vi "runTestScenario.vi"(0 "Constant Analog Output Voltage Test  in":refnum<class "Constant Analog Output Voltage Test.lvclass">, 5 "ILC":refnum<class "ILC.lvclass">, 11 "error in (no error)":errorcluster) -> (4 "Constant Analog Output Voltage Test  out":refnum<class "Constant Analog Output Voltage Test.lvclass">, 6 "ILC 2":refnum<class "ILC.lvclass">, 8 "TestExecution":T2, 10 "Result":T1, 15 "error out":errorcluster)   [LabVIEW 2016, in "Constant Analog Output Voltage Test.lvclass"]
uses:
  Constant Analog Output Voltage Test.lvclass
  Typedefs/TestExecution.ctl
  Typedefs/PassFailTest.ctl
  Common_ILC/ILC/ILC.lvclass
  Typedefs/WriteDataFileInput.ctl
  Typedefs/TestScenarioTypes.ctl
  Typedefs/WriteLogMessageInput.ctl
  Constant Analog Output Voltage Test.lvclass/Constant Analog Output Voltage Test.ctl
  Model/TestLog/ITestLog/ITestLog.lvclass
  Typedefs/ILCBTTypedefs.lvlib
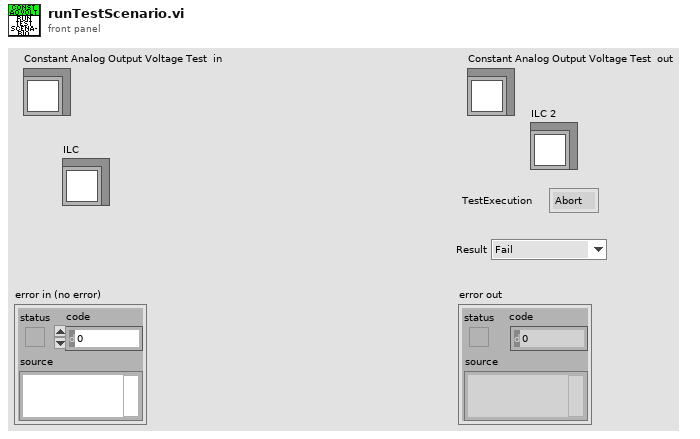
[diagram p1: front panel]
types:
  T1 = typedef "ILCBTTypedefs.lvlib/PassFailTest.ctl" = enum16{"Fail", "Pass", "NA"}
  T2 = typedef "ILCBTTypedefs.lvlib/TestExecution.ctl" = enum16{"Abort", "Continue"}
  T3 = typedef "ILCBTTypedefs.lvlib/WriteLogMessageInput.ctl" = cluster{"Test Scenario":T4, "Description":string, "Actual Value":string, "Data File":string, "Result":T1}
  T4 = typedef "ILCBTTypedefs.lvlib/TestScenarioTypes.ctl" = enum16{"+3.3VD", "+5.1V", "+24V", "RELVALV1", "RELVALV2", "Verify DAC_A = -1.00A", "Verify DAC_A = -0.75A", "Verify DAC_A = -0.50A", "Verify DAC_A = -0.25A", "Verify DAC_A = 0.00A", "Verify DAC_A = 0.25A", "Verify DAC_A = 0.50A", "Verify DAC_A = 0.75A", "Verify DAC_A = 1.00A", "Verify DAC_B = -1.00A", "Verify DAC_B = -0.75A", "Verify DAC_B = -0.50A", "Verify DAC_B = -0.25A", "Verify DAC_B = 0.00A", "Verify DAC_B = 0.25A", "Verify DAC_B = 0.50A", "Verify DAC_B = 0.75A", "Verify DAC_B = 1.00A", "Set DAC_A = -1.00A", "Set DAC_A = -0.75A", "Set DAC_A = -0.50A", "Set DAC_A = -0.25A", "Set DAC_A = 0.00A", "Set DAC_A = 0.25A", "Set DAC_A = 0.50A", "Set DAC_A = 0.75A", "Set DAC_A = 1.00A", "Set DAC_B = -1.00A", "Set DAC_B = -0.75A", "Set DAC_B = -0.50A", "Set DAC_B = -0.25A", "Set DAC_B = 0.00A", "Set DAC_B = 0.25A", "Set DAC_B = 0.50A", "Set DAC_B = 0.75A", "Set DAC_B = 1.00A", "Set MTR_PWR = On", "Set MTR_PWR = Off", "Set OUTPUT = On", "Set OUTPUT = Off", "Verify OUTPUT = On", "Verify OUTPUT = Off", "Verify POWER = Ok", "Verify POWER = Fail", "Verify AMP1 = Ok", "Verify AMP1 = Fail", "Verify AMP2 = Ok", "Verify AMP2 = Fail", "P1 0%", "P1 25%", "P1 50%", "P1 75%", "P1 100%", "P2 0%", "P2 25%", "P2 50%", "P2 75%", "P2 100%", "P3 0%", "P3 25%", "P3 50%", "P3 75%", "P3 100%", "P4 0%", "P4 25%", "P4 50%", "P4 75%", "P4 100%", "DCA 1 Linearity", "DCA 2 Linearity"}
  T5 = typedef "ILCBTTypedefs.lvlib/WriteDataFileInput.ctl" = cluster{"Test Scenario":T4, "File Name":string, "Output":string[]}
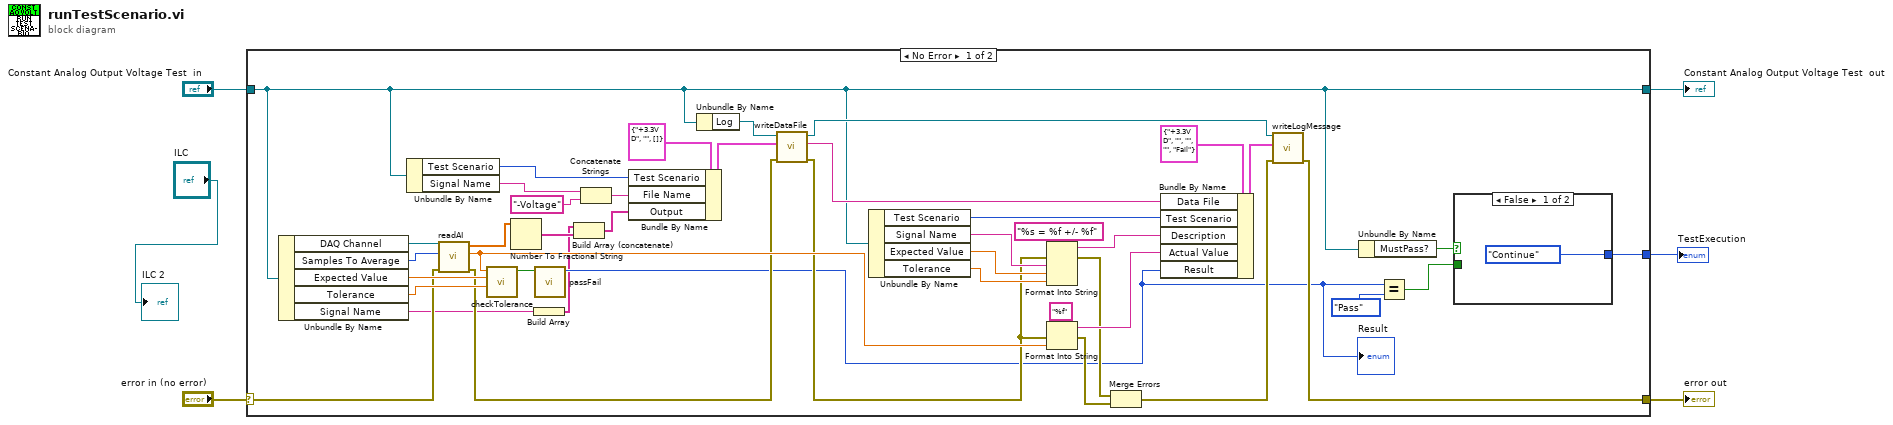
[diagram p0: block diagram]
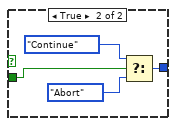
[diagram p2: hidden frame]
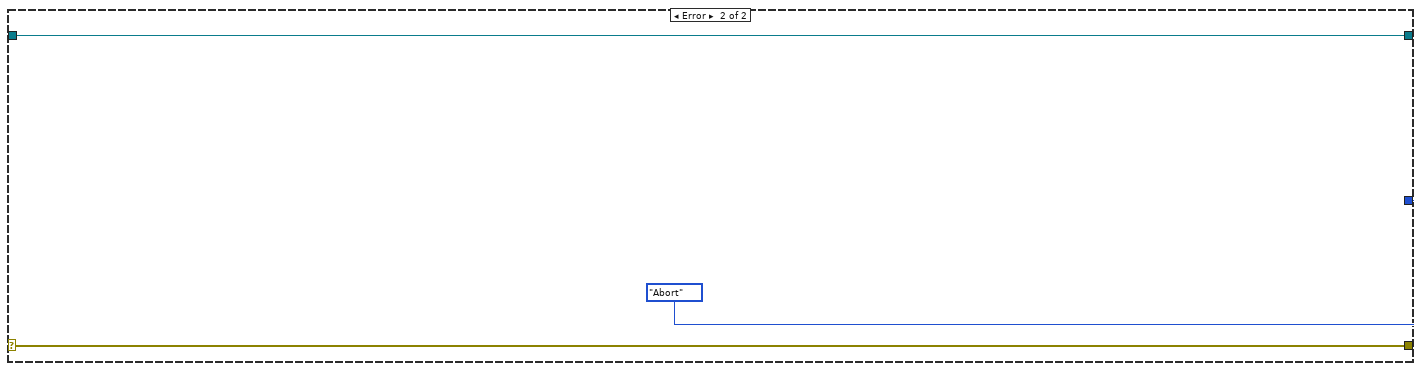
[diagram p3: hidden frame]
diagram:
  n1 = case shown="No Error" "error in (no error)" {
    selector: "error in (no error)" -> [w25 w57]
    tunnel: [w20 w57] -> w5
    tunnel: [w16 TestExecution."Abort" ("TestExecution")] -> w4
    tunnel: "Constant Analog Output Voltage Test  in" -> [w18 w55]
    tunnel: [w18 w55] -> w2
    frame No Error {
      n2 = Unbundle By Name(w18) -> ("DAQ Channel"=w49:refnum<k21>, "Samples To Average"=w42:i32, "Expected Value"=w41:dbl, "Tolerance"=w40:dbl, "Signal Name"=w8:string)
      n3 = Unbundle By Name(w18) -> ("Test Scenario"=w45:T4, "Signal Name"=w44:string)
      n4 = call "readAI.vi"("error in (no error)"=w25, "Samples To Read"=w42, "DAQ Channel To Read"=w49) -> ("error out"=w24:errorcluster, "Average"=w28:dbl, "Samples"=w13:dbl[])  [unwired: 6 in]
      n5 = call "checkTolerance.vi"("Tolerance"=w40, "Expected Value"=w41, "Average"=w28) -> ("Boolean"=w37:bool)  [unwired: 8 in]
      n6 = Number To Fractional String(number=w13) -> (F-format string=w10:string[])  [unwired: 3 in]
      n7 = Build Array(w8) -> (w7:string[])
      n8 = call "passFail.vi"("Boolean"=w37) -> ("Result"=w12:T1)  [unwired: 10 in]
      "Result" <- w12
      n9 = Build Array (concatenate)(w7, w10) -> (w9:string[])
      n10 = Concatenate Strings(w44, "-Voltage" ("string")) -> (w43:string)
      n11 = Bundle By Name(cluster=T5 {"Test Scenario"=enum."+3.3VD", "File Name"="", "Output"=[]} ("WriteDataFileInput"), "Test Scenario"=w45, "File Name"=w43, "Output"=w9) -> (w46:T5)
      n12 = Unbundle By Name(w18) -> ("Log"=w48:refnum<class "ITestLog.lvclass">)
      n13 = call-dynamic "writeDataFile.vi"("error in (no error)"=w24, "WriteDataFileInput"=w46, "ITestLog in"=w48) -> ("error out"=w19:errorcluster, "Relative Path"=w36:string, "ITestLog out"=w26:refnum<class "ITestLog.lvclass">)  [unwired: 6 in]
      n14 = Unbundle By Name(w18) -> ("Test Scenario"=w35:T4, "Signal Name"=w33:string, "Expected Value"=w32:dbl, "Tolerance"=w31:dbl)
      n15 = Format Into String(format string="%s = %f +/- %f", error in=w19, w33, w32, w31) -> (resulting string=w30:string, error out=w23:errorcluster)  [unwired: 1 in]
      n16 = Format Into String(format string="%f", error in=w19, w28) -> (resulting string=w27:string, error out=w22:errorcluster)  [unwired: 1 in]
      n17 = Merge Errors(w23, w22) -> (w21:errorcluster)
      n18 = Bundle By Name(cluster=T3 {"Test Scenario"=enum."+3.3VD", "Description"="", "Actual Value"="", "Data File"="", "Result"=enum."Fail"} ("WriteLogMessageInput"), "Data File"=w36, "Test Scenario"=w35, "Description"=w30, "Actual Value"=w27, "Result"=w12) -> (w38:T3)
      n19 = call-dynamic "writeLogMessage.vi"("error in (no error)"=w21, "WriteLogMessageInput"=w38, "ITestLog in"=w26) -> ("error out"=w20:errorcluster)  [unwired: 7 in, 1 out]
      n20 = Unbundle By Name(w18) -> ("MustPass?"=w17:bool)
      n21 = Equal?(x=w12, y=PassFailTest."Pass") -> (x = y?=w14:bool)
      n22 = case shown="False" w17 {
        tunnel: [TestExecution."Continue" ("TestExecution") w54] -> w16
        tunnel: w14 -> [_ w51]
        frame False {
        }
        frame True {
          n23 = Select(t=TestExecution."Continue" ("TestExecution"), s=w51, f=TestExecution."Abort" ("TestExecution")) -> (s? t:f=w54:T2)
        }
      }
    }
    frame Error {
    }
  }
  "Constant Analog Output Voltage Test  out" <- w2
  "error out" <- w5
  "TestExecution" <- w4
  "ILC 2" <- "ILC"
